vi "Destroy Event Registrations.vi"(8 "error in (no error)":errorcluster, 11 "Event-Registrations":T1) -> (0 "error out":errorcluster)   [LabVIEW 2018, in "Copy of Actor.lvclass"]
uses:
  Copy of Actor.lvclass
  Event-Registrations.ctl
  Stop.ctl
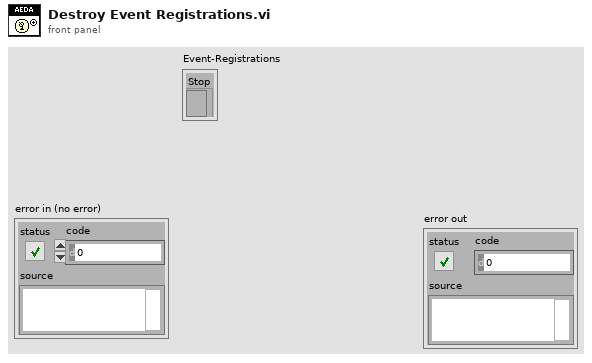
[diagram p1: front panel]
types:
  T1 = typedef "Copy of Actor.lvclass/Event-Registrations.ctl" = cluster{"Stop":refnum<event-registration>}
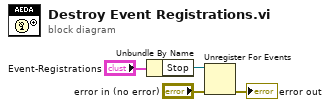
[diagram p0: block diagram]
diagram:
  n1 = Unbundle By Name("Event-Registrations") -> ("Stop"=w3:refnum<event-registration>)
  n2 = Unregister For Events(event registration refnum=w3, error in="error in (no error)") -> (error out=→"error out":errorcluster)
